vi "XIPIN_AXI_Data_Width_Converter_2_1.vi"   [LabVIEW 2017]
doc: "The AXI Data Width Converter IP provides the facility to increase or decrease the data width of WDATA and RDATA between an AXI4/AXI3/AXI4-Lite master and slave.\n------------------------------------\n<b>Need License</b> : No\n<b>Interface</b> : AXI4"
uses:
  <vilib>/rvi/XilinxIP/XIPIN_XNode/niFpgaXIPIN.xnode
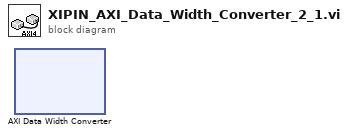
[diagram p0: block diagram]
diagram:
  n1 = xnode ("AXI Data Width Converter")() -> ()
